vi "Cobra_Front_Panel_Basic.vi"() -> ()   [LabVIEW 2015]
panel:
  in  "RESET Button":bool
  in  "Internal Trigger":bool=TRUE
  in  "EXIT":bool
  in  "Line Scan Enable":bool=TRUE
  in  "Line Time Value":u16=90 step=1
  in  "Integration Time Value":u16=100 min=1 max=32767 step=1
  in  "Offset Value":u16=255 max=255 step=1
  in  "Gain Value":u16=187 max=255 step=1
  out "Configuration String Sent":string
  out "Failure":bool
  out "Initialized":bool
  in  "Set":bool
  out "Characters Read":u32
  out "IMAQ Session Out":refnum<k11>
  out "Command Data Read":string
  out "Error Output":errorcluster
  in  "error in (no error)":errorcluster
  # "Suggested Starting Values:\n\nGain: 187\nOffset: 255\nIntegration Time: 90\nLine Time: 100"
  # "Inital Setup and Connection:\n\n  1. Launch NI MAX, select the camera (should be img0).\n  2. Load the supplied *.icd file for the camera.\n  3. Close NI MAX.\n  4. Run this VI and click the \"Set all\" button."
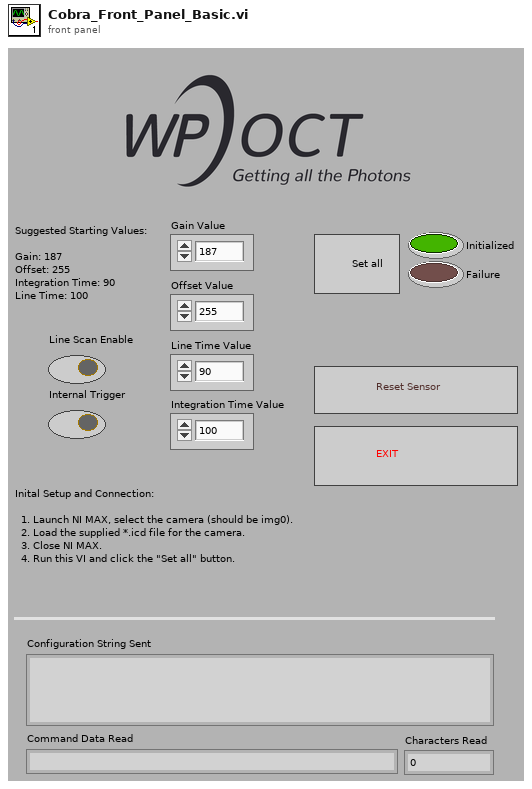
[diagram p1: front panel]
types:
  T1 = typedef "imagedata.ctl" = cluster{"image type":i32, "image depth":i32, "image":u8[], "mask":u8[], "colors":u32[], "Rectangle":cluster{"left":i16, "top":i16, "right":i16, "bottom":i16}}
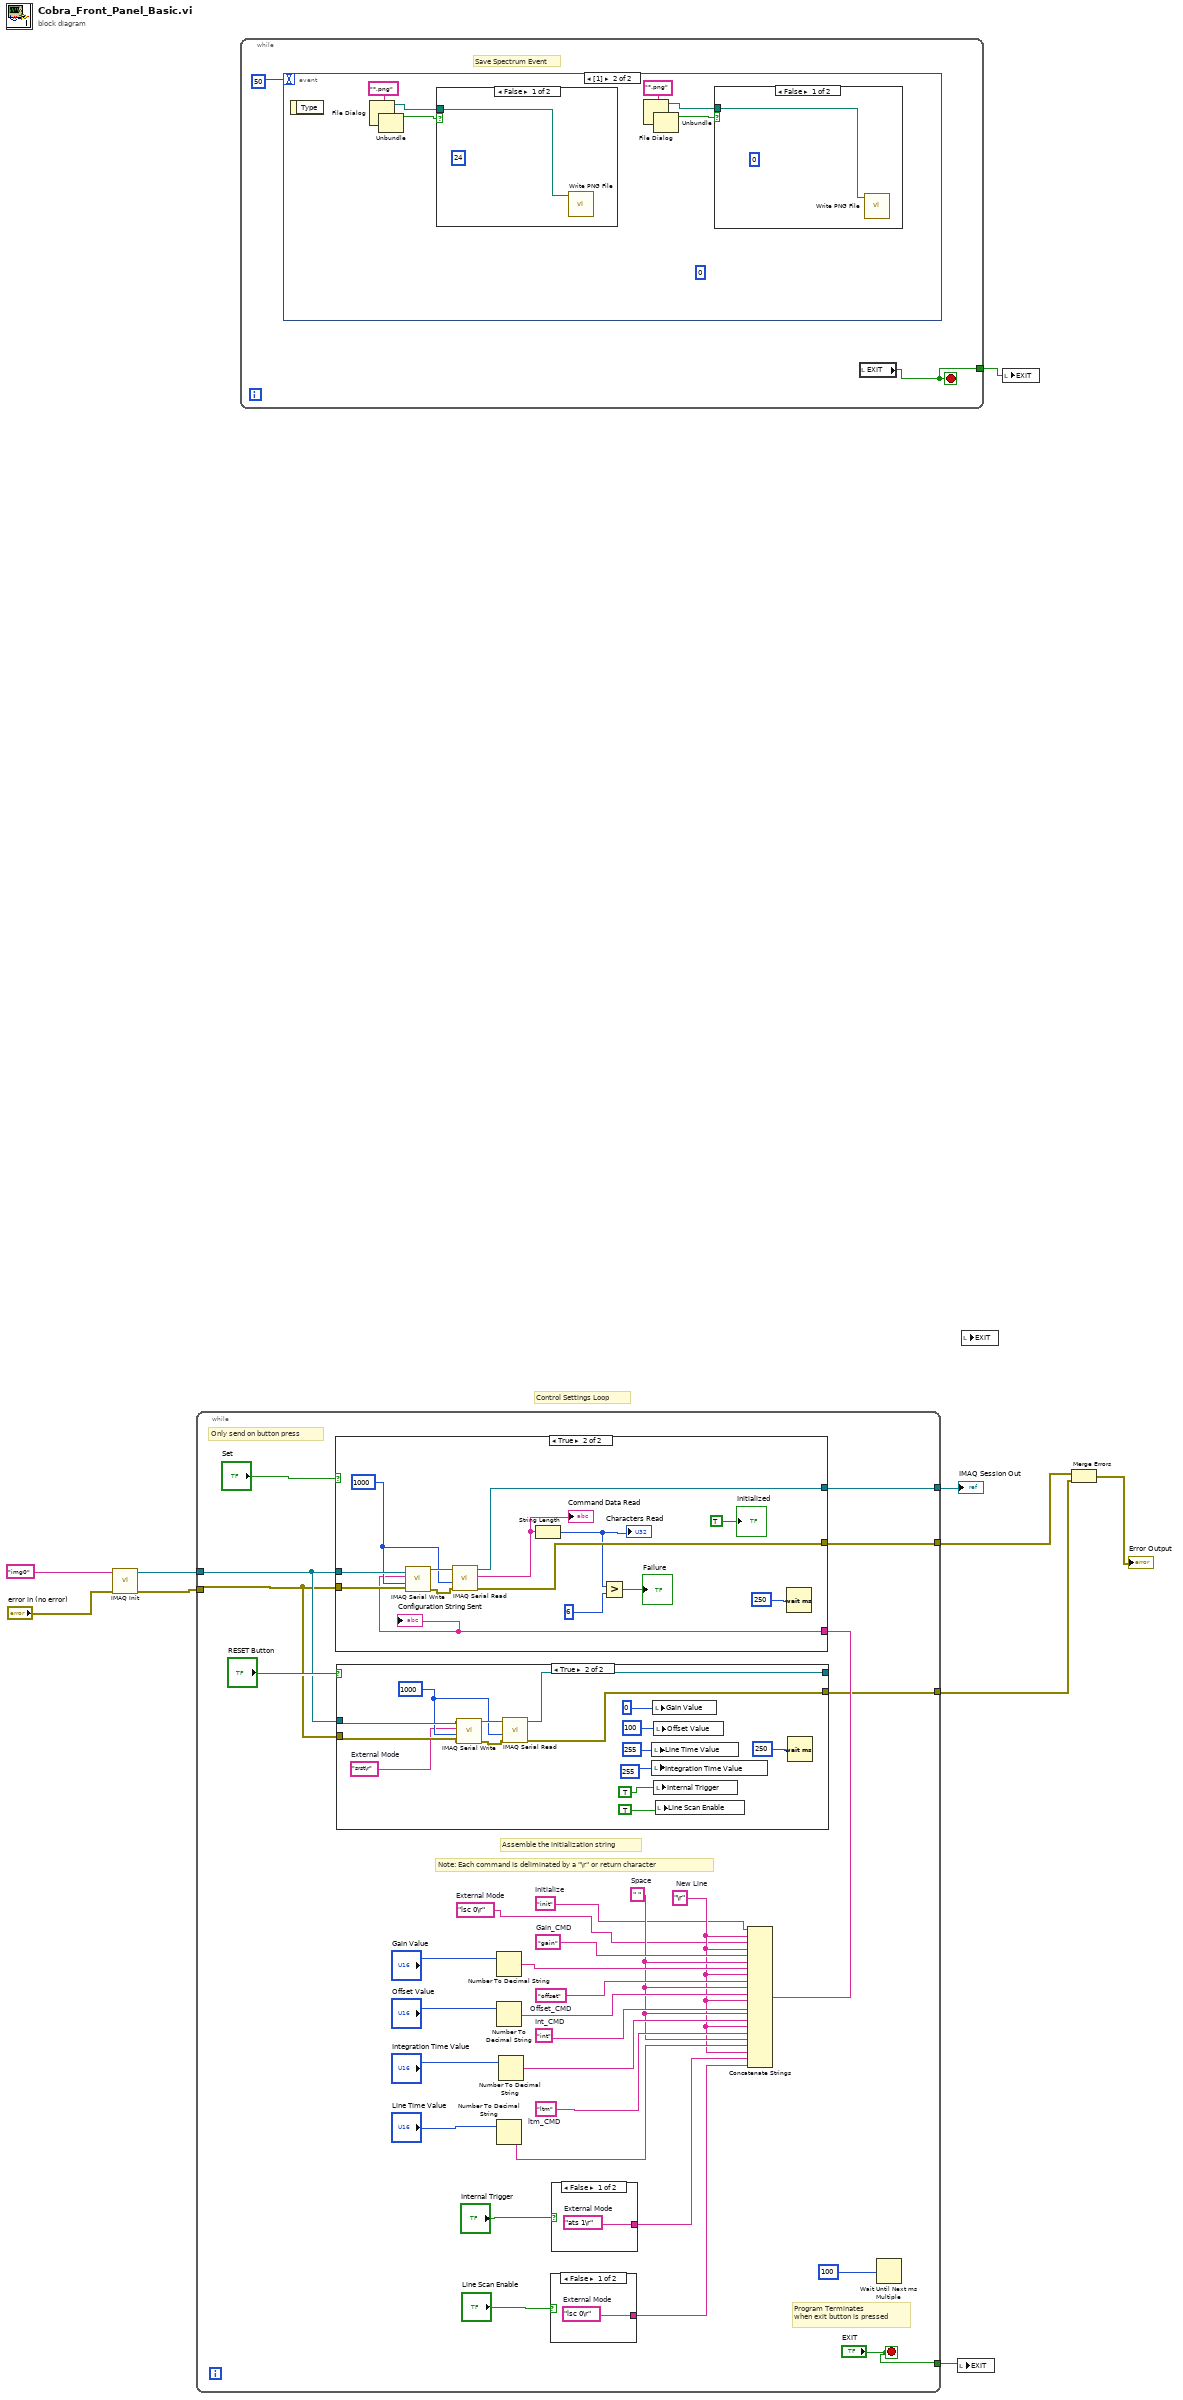
[diagram p0: block diagram]
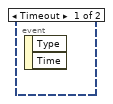
[diagram p2: hidden frame]
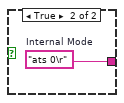
[diagram p6: hidden frame]
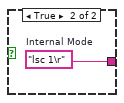
[diagram p8: hidden frame]
diagram:
  # "Control Settings Loop"
  n1 = call <vilib>:"IMAQ Init.vi"("error in (no error)"="error in (no error)", "Interface Name"="img0") -> ("error out"=w7:errorcluster, "IMAQ Session Out"=w8:refnum<k11>)  [unwired: 8 in]
  n2 = while {
    tunnel: w8 -> [w14]
    tunnel: w7 -> [w13]
    tunnel: [w40] -> w9
    tunnel: [w39] -> w6
    tunnel: [w12] -> w3
    tunnel: ["EXIT"] -> w2
    stop <- "EXIT" stop-if-true
    w20 = "lsc 0\r"  # External Mode
    w28 = "ltm"  # ltm_CMD
    w27 = "int"  # Int_CMD
    w26 = "offset"  # Offset_CMD
    w25 = "gain"  # Gain_CMD
    w22 = " "  # Space
    w21 = "\r"  # New Line
    w19 = "init"  # Initialize
    # "Program Terminates\nwhen exit button is pressed"
    # "Only send on button press"
    # "Note: Each command is deliminated by a \"\\r\" or return character"
    # "Assemble the initialization string"
    n3 = case shown="True" "RESET Button" {
      tunnel: w14 -> [w42 w52]
      tunnel: w13 -> [w41 w50]
      tunnel: [w42 w57] -> _
      tunnel: [w41 w56] -> w12
      frame False {
      }
      frame True {
        w49 = "srst\r"  # External Mode
        w51 = 1000
        n4 = call <vilib>:"IMAQ Serial Write.vi"("error in (no error)"=w50, "Timeout"=w51, "String to write"=w49, "IMAQ Session In"=w52) -> ("error out"=w53:errorcluster, "IMAQ Session Out"=w54:refnum<k11>)  [unwired: 4 in]
        n5 = call <vilib>:"IMAQ Serial Read.vi"("error in (no error)"=w53, "Timeout"=w51, "IMAQ Session In"=w54) -> ("error out"=w56:errorcluster, "IMAQ Session Out"=w57:refnum<k11>)  [unwired: 3 in, 2 out]
        n6 = local write "Line Time Value"(255) -> ()
        n7 = local write "Integration Time Value"(255) -> ()
        n8 = local write "Gain Value"(0) -> ()
        n9 = local write "Offset Value"(100) -> ()
        n10 = local write "Internal Trigger"(TRUE) -> ()
        n11 = local write "Line Scan Enable"(TRUE) -> ()
        n12 = Wait (ms)(milliseconds to wait=250) -> ()  [unwired: 1 out]
      }
    }
    n13 = Number To Decimal String(number="Gain Value") -> (decimal integer string=w29:string)  [unwired: 1 in]
    n14 = Number To Decimal String(number="Offset Value") -> (decimal integer string=w31:string)  [unwired: 1 in]
    n15 = Number To Decimal String(number="Line Time Value") -> (decimal integer string=w36:string)  [unwired: 1 in]
    n16 = Number To Decimal String(number="Integration Time Value") -> (decimal integer string=w34:string)  [unwired: 1 in]
    n17 = case shown="False" "Line Scan Enable" {
      tunnel: [w76 w77] -> w16
      frame False {
        w76 = "lsc 0\r"  # External Mode
      }
      frame True {
        w77 = "lsc 1\r"  # Internal Mode
      }
    }
    n18 = case shown="False" "Internal Trigger" {
      tunnel: [w58 w59] -> w17
      frame False {
        w58 = "ats 1\r"  # External Mode
      }
      frame True {
        w59 = "ats 0\r"  # Internal Mode
      }
    }
    n19 = Concatenate Strings(w19, w21, w20, w21, w25, w22, w29, w21, w26, w22, w31, w21, w27, w22, w34, w21, w28, w22, w36, w21, w17, w16) -> (w24:string)
    n20 = case shown="True" "Set" {
      tunnel: w14 -> [w61 w69]
      tunnel: w13 -> [w60 w67]
      tunnel: [w61 w75] -> w40
      tunnel: [w60 w74] -> w39
      tunnel: w24 -> [_ w66]
      frame False {
      }
      frame True {
        w68 = 1000
        n21 = call <vilib>:"IMAQ Serial Write.vi"("error in (no error)"=w67, "Timeout"=w68, "String to write"=w66, "IMAQ Session In"=w69) -> ("error out"=w70:errorcluster, "IMAQ Session Out"=w71:refnum<k11>)  [unwired: 4 in]
        n22 = call <vilib>:"IMAQ Serial Read.vi"("error in (no error)"=w70, "Timeout"=w68, "IMAQ Session In"=w71) -> ("error out"=w74:errorcluster, "String Read"=w65:string, "IMAQ Session Out"=w75:refnum<k11>)  [unwired: 3 in, 1 out]
        "Command Data Read" <- w65
        n23 = String Length(string=w65) -> (length=w64:i32)
        "Characters Read" <- w64
        n24 = Greater?(x=w64, y=6) -> (0:→"Failure":bool)
        n25 = Wait (ms)(milliseconds to wait=250) -> ()  [unwired: 1 out]
        "Configuration String Sent" <- w66
        "Initialized" <- TRUE
      }
    }
    n26 = Wait Until Next ms Multiple(millisecond multiple=100) -> ()  [unwired: 1 out]
  }
  "IMAQ Session Out" <- w9
  n27 = while {
    tunnel: [w79] -> w1
    stop <- w79 stop-if-true
    # "Save Spectrum Event"
    n28 = event shown="[1]" {
      selector: _ -> [_ _]
      dyn-events: _ -> [_ _]
      timeout: 50 -> [_ _]
      event Timeout {
        n29 = event-data() -> ()  [unwired: 1 in, 2 out]
      }
      event #1 (no event record) {
        w80 = 0 ("image depth")
        n30 = event-data() -> ()  [unwired: 1 in, 1 out]
        n31 = File Dialog(6:"*.png" ("pattern")) -> (0:w88:errorcluster, 1:w86:bool, 3:w85:path)  [unwired: 6 in, 1 out]
        n32 = Unbundle(w88) -> ()  [unwired: 3 out]
        n33 = case shown="False" w86 {
          tunnel: w85 -> [w93 _]
          frame False {
            w92 = 24 ("image depth")
            n34 = call <vilib>:"Write PNG File.vi"("path to PNG file"=w93) -> ("image data"=w91:T1)  [unwired: 8 in, 2 out]
          }
          frame True {
          }
        }
        n35 = File Dialog(6:"*.png" ("pattern")) -> (0:w84:errorcluster, 1:w82:bool, 3:w81:path)  [unwired: 6 in, 1 out]
        n36 = Unbundle(w84) -> ()  [unwired: 3 out]
        n37 = case shown="False" w82 {
          tunnel: w81 -> [w90 _]
          frame False {
            (unwired) 0 ("image depth")
            n38 = call <vilib>:"Write PNG File.vi"("path to PNG file"=w90) -> ("image data"=w89:T1)  [unwired: 8 in, 2 out]
          }
          frame True {
          }
        }
      }
    }
    n39 = local read "EXIT"() -> (w79:bool)
  }
  n40 = local write "EXIT"(w2) -> ()
  n41 = local read "EXIT"() -> ()  [unwired: 1 in]
  n42 = local write "EXIT"(w1) -> ()
  n43 = Merge Errors(w6, w3) -> (→"Error Output":errorcluster)
